vi "File Popup For Load.vi"(8 "error in (no error)":errorcluster) -> (0 "error out":errorcluster, 2 "cancelled":bool, 3 "selected path":path)   [LabVIEW 2021]
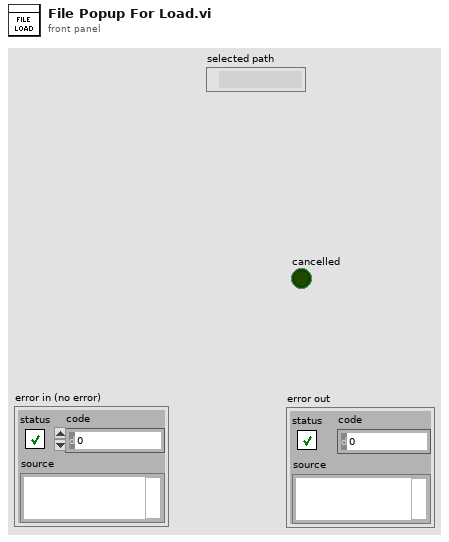
[diagram p1: front panel]
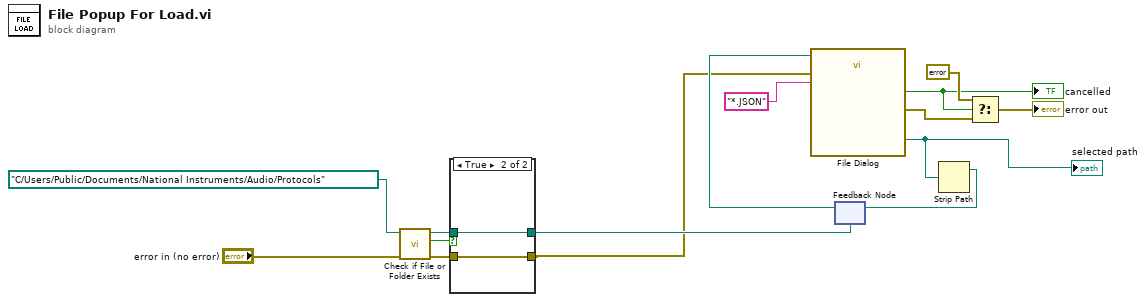
[diagram p0: block diagram]
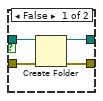
[diagram p2: hidden frame]
diagram:
  n1 = call <vilib>:"Check if File or Folder Exists.vi"("error in (no error)"="error in (no error)", "path"=path "C:/Users/Public/Documents/National Instruments/Audio/Protocols") -> ("error out"=w14:errorcluster, "file or folder exists?"=w15:bool, "dup path"=w13:path)  [unwired: 7 in]
  n2 = case shown="True" w15 {
    tunnel: w14 -> [w19 w20]
    tunnel: w13 -> [w18 w21]
    tunnel: [w17 w21] -> w10
    tunnel: [w16 w20] -> w5
    frame False {
      n3 = Create Folder(path (use dialog)=w18, error in=w19) -> (created path=w17:path, error out=w16:errorcluster)  [unwired: 1 in, 1 out]
    }
    frame True {
    }
  }
  n4 = feedback #1(w10) -> (w6:path)
  n5 = call "File Dialog"("start path"=w6, "error in"=w5, "pattern (all files)"="*.JSON") -> ("selected path"=w1:path, "cancelled"=w3:bool, "error out"=w2:errorcluster)  [unwired: 9 in, 1 out]
  "cancelled" <- w3
  "selected path" <- w1
  n6 = Strip Path(path=w1) -> (stripped path=w11:path)  [unwired: 1 out]
  n7 = feedback-in #1(w11) -> ()
  n8 = Select(t=errorcluster {"status"=FALSE, "code"=0, "source"=""}, s=w3, f=w2) -> (s? t:f=→"error out":errorcluster)
